vi "Cleanup.vi"(8 "error in (no error)":errorcluster, 11 "DeviceManager in":refnum<class "DeviceManager.lvclass">) -> (0 "error out":errorcluster)   [LabVIEW 2020, in "PicoG-Core.lvlib" / "DeviceManager.lvclass"]
uses:
  DeviceManager.lvclass
  DeviceManager.lvclass/DeviceManager.ctl
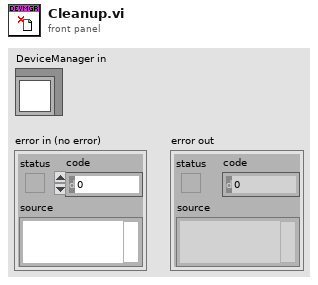
[diagram p1: front panel]
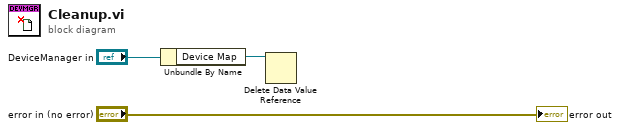
[diagram p0: block diagram]
diagram:
  n1 = Unbundle By Name("DeviceManager in") -> ("Device Map"=w1:refnum<data-value>)
  n2 = Delete Data Value Reference(data value reference=w1) -> ()  [unwired: 1 in, 2 out]
  "error out" <- "error in (no error)"
